vi "Get KF Observer.vi"(8 "error in (no error)":errorcluster, 11 "Vessel in":refnum<class "Vessel.lvclass">) -> (0 "error out":errorcluster, 2 "Active Observer":refnum<class "Observer.lvclass">, 3 "Vessel out":refnum<class "Vessel.lvclass">)   [LabVIEW 2014, in "Vessel.lvclass"]
uses:
  Vessel.lvclass
  Observer/Observer.lvclass
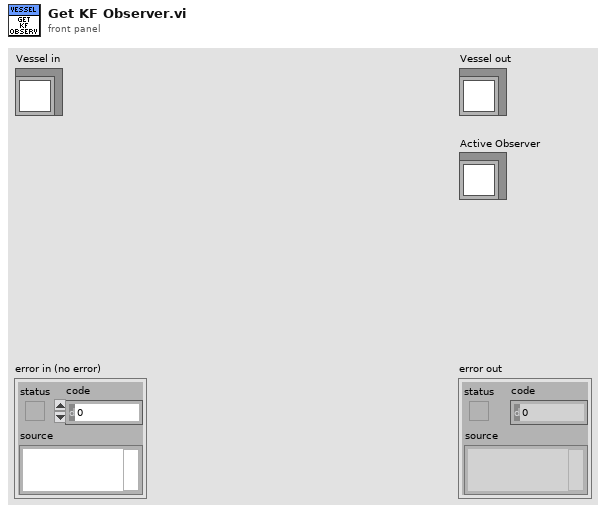
[diagram p1: front panel]
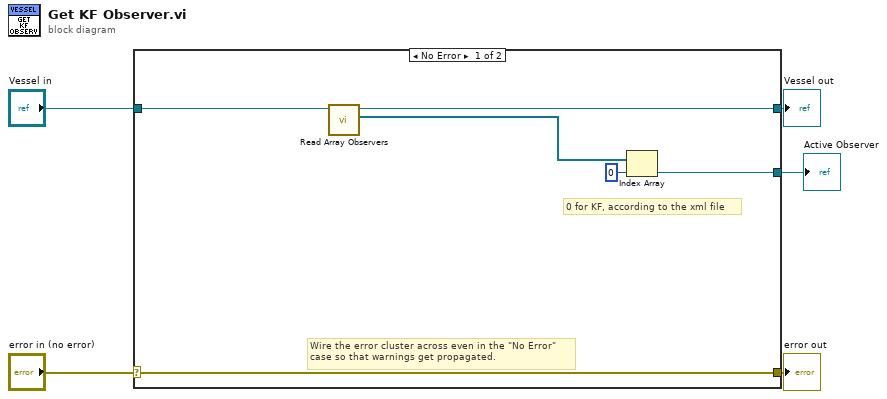
[diagram p0: block diagram]
diagram:
  n1 = case shown="No Error" "error in (no error)" {
    selector: "error in (no error)" -> [w11 w13]
    tunnel: [w11 w13] -> w4
    tunnel: [w10 w12] -> w2
    tunnel: "Vessel in" -> [w9 w12]
    tunnel: [w7 _] -> w1
    frame No Error {
      # "0 for KF, according to the xml file"
      # "Wire the error cluster across even in the \"No Error\"\ncase so that warnings get propagated."
      n2 = call-dynamic "Read Array Observers.vi"("Vessel in"=w9) -> ("Array Observers"=w8:refnum<class "Observer.lvclass">[], "Vessel out"=w10:refnum<class "Vessel.lvclass">)  [unwired: 8 in, 1 out]
      n3 = Index Array(array=w8, index=0) -> (element=w7:refnum<class "Observer.lvclass">)
    }
    frame Error {
    }
  }
  "error out" <- w4
  "Vessel out" <- w2
  "Active Observer" <- w1
